vi "Tag Find2.vi"(0 "Tree Reference In":refnum<vi>, 2 "Input Text":string, 5 "error in (no error)":errorcluster) -> (14 "Tree Reference Out":refnum<vi>, 16 "Duplicate Text":string, 17 "Text Tag":string, 19 "error out":errorcluster)   [LabVIEW 2014]
doc: "Searches the tree for a tag whose text matches the Input text.\n \nUSE SPARINGLY - Processor Intensive"
panel:
  in  "Column # (0)":i32
  # "VI INPUTS"
  # "VI OUTPUTS"
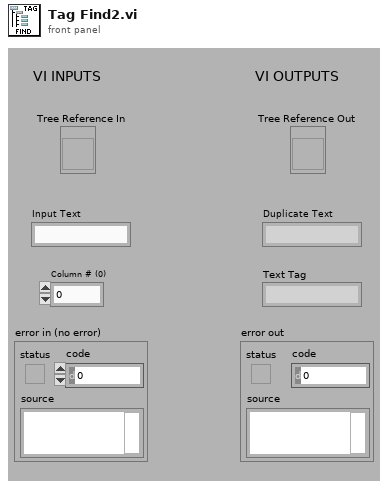
[diagram p1: front panel]
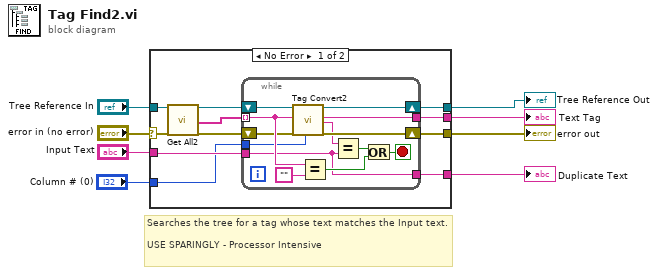
[diagram p0: block diagram]
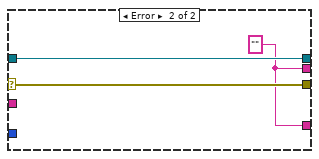
[diagram p2: hidden frame]
diagram:
  # "Searches the tree for a tag whose text matches the Input text.\n \nUSE SPARINGLY - Processor Intensive"
  n1 = case shown="No Error" "error in (no error)" {
    tunnel: "Tree Reference In" -> [w19 w35]
    selector: "error in (no error)" -> [w18 w34]
    tunnel: [w10 w35] -> w8
    tunnel: [w13 w34] -> w7
    tunnel: "Input Text" -> [w15 _]
    tunnel: [w12 w33] -> w3
    tunnel: [w11 w33] -> w2
    tunnel: "Column # (0)" -> [w9 _]
    frame No Error {
      n2 = call "Get All2.vi"("Tree Reference In"=w19, "error in (no error)"=w18) -> ("Tree Reference Out"=w16:refnum<vi>, "Output Tree Items"=w17:string[], "error out"=w14:errorcluster)  [unwired: 14 in, 1 out]
      n3 = while {
        tunnel: w17 -> [w30] mode=indexing
        shift-right: [w26] -> w10
        shift-left: w16 -> [w32]
        tunnel: w15 -> [w23]
        shift-right: [w24] -> w13
        shift-left: w14 -> [w25]
        tunnel: [w21] -> w11
        tunnel: [w23] -> w12
        tunnel: w9 -> [w20]
        stop <- w27 stop-if-true
        n4 = call "Tag Convert2.vi"("Tree Reference In"=w32, "InputTag (Current)"=w30, "error in (no error)"=w25, "Column # (0)"=w20) -> ("Tree Reference Out"=w26:refnum<vi>, "Duplicate Tag"=w21:string, "Tag Text"=w22:string, "error out"=w24:errorcluster)  [unwired: 12 in]
        n5 = Equal?(x=w30, y="") -> (x = y?=w28:bool)
        n6 = Equal?(x=w22, y=w23) -> (x = y?=w31:bool)
        n7 = Or(x=w31, y=w28) -> (x .or. y?=w27:bool)
      }
    }
    frame Error {
      w33 = ""
    }
  }
  "Tree Reference Out" <- w8
  "error out" <- w7
  "Text Tag" <- w2
  "Duplicate Text" <- w3
